vi "Cell detection grassfire.vi"(1 "Intensities":u8[][](array[numeric])) -> (0 "Cell":u8[][](array[numeric]))   [LabVIEW 2019]
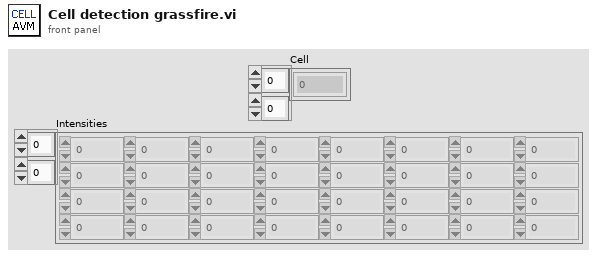
[diagram p1: front panel]
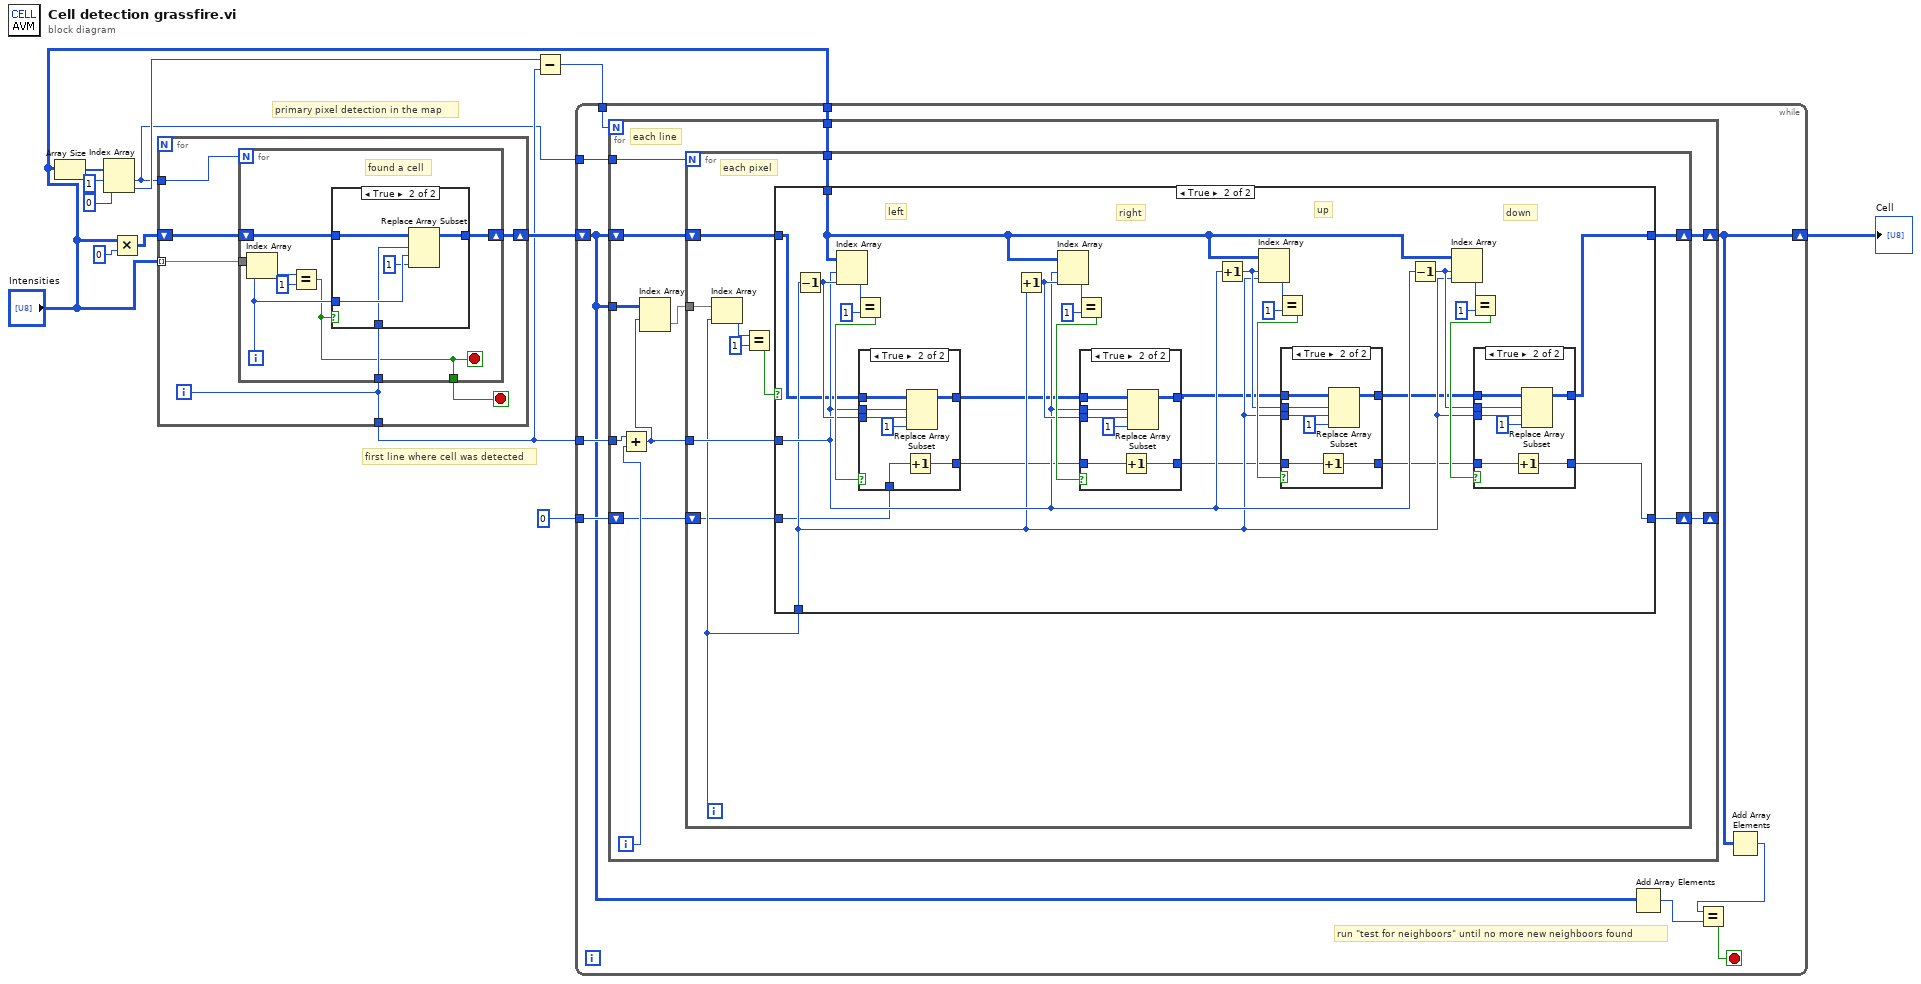
[diagram p0: block diagram]
diagram:
  # "first line where cell was detected"
  # "primary pixel detection in the map"
  n1 = Array Size(array="Intensities") -> (size(s)=w12:i32[])
  n2 = Index Array(array=w12, index #1=1 ("y"), index #2=0 ("y")) -> (element #1=w1:i32, element #2=w2:i32)
  n3 = Multiply(x="Intensities", y=i16 0) -> (x*y=w10:i16[][])
  n4 = for {
    tunnel: w1 -> [w19]
    tunnel: "Intensities" -> [w18] mode=indexing
    shift-right: [w16] -> w9
    shift-left: w10 -> [w17]
    tunnel: [w14] -> w6
    i -> [w14]
    stop <- w15 stop-if-true
    n5 = for {
      N: w19 -> [_]
      tunnel: w18 -> [w27]
      tunnel: w14 -> [w22]
      shift-right: [w23] -> w16
      shift-left: w17 -> [w24]
      tunnel: [w20] -> w15
      i -> [w21]
      stop <- w20 stop-if-true
      # "found a cell"
      n6 = Index Array(array=w27, index=w21) -> (element=w25:u8)
      n7 = Equal?(x=w25, y=i16 1) -> (x = y?=w20:bool)
      n8 = case shown="True" w20 {
        tunnel: w24 -> [w28 w29]
        tunnel: w21 -> [_ w33]
        tunnel: w22 -> [_ w32]
        tunnel: [w28 w30] -> w23
        frame False {
        }
        frame True {
          n9 = Replace Array Subset(array=w29, new element=i16 1 ("y"), index (row)=w32, index (col)=w33) -> (w30:i16[][])
        }
      }
    }
  }
  n10 = Subtract(x=w2, y=w6) -> (x-y=w7:i32)
  n11 = while {
    tunnel: w6 -> [w43]
    shift-right: [w37] -> w3
    shift-left: w9 -> [w36]
    tunnel: w1 -> [w42]
    tunnel: w7 -> [w41]
    tunnel: i16 0 ("y") -> [w40]
    tunnel: "Intensities" -> [w39]
    stop <- w38 stop-if-true
    # "run \"test for neighboors\" until no more new neighboors found"
    n12 = for {
      N: w41 -> [_]
      shift-right: [w51] -> w37
      shift-left: w36 -> [w54]
      tunnel: w43 -> [w53]
      tunnel: w36 -> [w49]
      tunnel: w42 -> [w50]
      shift-right: [w46] -> _
      shift-left: w40 -> [w45]
      tunnel: w39 -> [w44]
      i -> [w52]
      # "each line"
      n13 = Add(x=w53, y=w52) -> (x+y=w48:i32)
      n14 = Index Array(array=w49, index (row)=w48) -> (element=w47:i16[])  [unwired: 1 in]
      n15 = for {
        N: w50 -> [_]
        shift-right: [w59] -> w51
        shift-left: w54 -> [w65]
        tunnel: w48 -> [w64]
        tunnel: w47 -> [w60]
        shift-right: [w57] -> w46
        shift-left: w45 -> [w56]
        tunnel: w44 -> [w55]
        i -> [w58]
        # "each pixel"
        n16 = Index Array(array=w60, index=w58) -> (element=w62:i16)
        n17 = Equal?(x=w62, y=1) -> (x = y?=w61:bool)
        n18 = case shown="True" w61 {
          tunnel: w65 -> [w67 w73]
          tunnel: w64 -> [_ w81]
          tunnel: w58 -> [_ w79]
          tunnel: [w67 w70] -> w59
          tunnel: [w66 w74] -> w57
          tunnel: w56 -> [w66 w78]
          tunnel: w55 -> [_ w72]
          frame False {
          }
          frame True {
            # "down"
            # "up"
            # "right"
            # "left"
            n19 = Decrement(x=w79) -> (x-1=w93:i32)
            n20 = Index Array(array=w72, index (row)=w81, index (col)=w93) -> (element=w95:u8)
            n21 = Equal?(x=w95, y=1) -> (x = y?=w94:bool)
            n22 = case shown="True" w94 {
              tunnel: w73 -> [w125 w131]
              tunnel: [w125 w132] -> w71
              tunnel: w81 -> [_ w130]
              tunnel: w93 -> [_ w129]
              tunnel: w78 -> [w124 w127]
              tunnel: [w124 w126] -> w77
              frame False {
              }
              frame True {
                n23 = Increment(x=w127) -> (x+1=w126:i16)
                n24 = Replace Array Subset(array=w131, new element=i16 1 ("y"), index (row)=w130, index (col)=w129) -> (w132:i16[][])
              }
            }
            n25 = Increment(x=w79) -> (x+1=w89:i32)
            n26 = Index Array(array=w72, index (row)=w81, index (col)=w89) -> (element=w91:u8)
            n27 = Equal?(x=w91, y=1) -> (x = y?=w90:bool)
            n28 = case shown="True" w90 {
              tunnel: w71 -> [w116 w122]
              tunnel: [w116 w123] -> w69
              tunnel: w81 -> [_ w121]
              tunnel: w89 -> [_ w120]
              tunnel: w77 -> [w115 w117]
              tunnel: [w115 w118] -> w76
              frame False {
              }
              frame True {
                n29 = Increment(x=w117) -> (x+1=w118:i16)
                n30 = Replace Array Subset(array=w122, new element=i16 1 ("y"), index (row)=w121, index (col)=w120) -> (w123:i16[][])
              }
            }
            n31 = Increment(x=w81) -> (x+1=w82:i32)
            n32 = Index Array(array=w72, index (row)=w82, index (col)=w79) -> (element=w87:u8)
            n33 = Equal?(x=w87, y=1) -> (x = y?=w86:bool)
            n34 = case shown="True" w86 {
              tunnel: w69 -> [w107 w113]
              tunnel: [w107 w114] -> w68
              tunnel: w82 -> [_ w112]
              tunnel: w79 -> [_ w111]
              tunnel: w76 -> [w106 w109]
              tunnel: [w106 w108] -> w75
              frame False {
              }
              frame True {
                n35 = Increment(x=w109) -> (x+1=w108:i16)
                n36 = Replace Array Subset(array=w113, new element=i16 1 ("y"), index (row)=w112, index (col)=w111) -> (w114:i16[][])
              }
            }
            n37 = Decrement(x=w81) -> (x-1=w80:i32)
            n38 = Index Array(array=w72, index (row)=w80, index (col)=w79) -> (element=w84:u8)
            n39 = Equal?(x=w84, y=1) -> (x = y?=w83:bool)
            n40 = case shown="True" w83 {
              tunnel: w68 -> [w98 w104]
              tunnel: [w98 w105] -> w70
              tunnel: w80 -> [_ w103]
              tunnel: w79 -> [_ w102]
              tunnel: w75 -> [w97 w99]
              tunnel: [w97 w100] -> w74
              frame False {
              }
              frame True {
                n41 = Increment(x=w99) -> (x+1=w100:i16)
                n42 = Replace Array Subset(array=w104, new element=i16 1 ("y"), index (row)=w103, index (col)=w102) -> (w105:i16[][])
              }
            }
          }
        }
      }
    }
    n43 = Add Array Elements(numeric array=w36) -> (sum=w34:i16)
    n44 = Add Array Elements(numeric array=w37) -> (sum=w35:i16)
    n45 = Equal?(x=w35, y=w34) -> (x = y?=w38:bool)
  }
  "Cell" <- w3
